vi "FlatToRichniswitch_grpc_GetErrorResponse.vi"(5 "OutputClusterType":T1, 11 "InputCluster":T2) -> (3 "OutputCluster":T1)   [LabVIEW 2021, in "NI Switch_client.lvlib"]
uses:
  NI Switch_client.lvlib
  niswitch_grpc_GetErrorResponse_Flat.ctl
  niswitch_grpc_GetErrorResponse.ctl
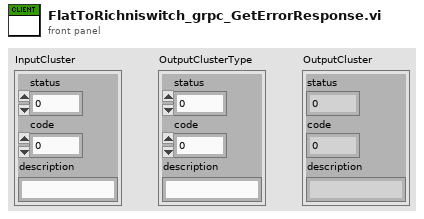
[diagram p1: front panel]
types:
  T1 = typedef "NI Switch_client.lvlib/niswitch_grpc_GetErrorResponse.ctl" = cluster{"status":i32, "code":i32, "description":string}
  T2 = typedef "NI Switch_client.lvlib/niswitch_grpc_GetErrorResponse_Flat.ctl" = cluster{"status":i32, "code":i32, "description":string}
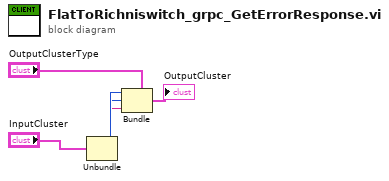
[diagram p0: block diagram]
diagram:
  n1 = Unbundle "Unbundle"("InputCluster") -> ("status"=w3:i32, "code"=w2:i32, "description"=w1:string)
  n2 = Bundle "Bundle"(cluster="OutputClusterType", "status"=w3, "code"=w2, "description"=w1) -> (→"OutputCluster":T1)
